vi "05T_Close_connection.vi"(11 "VISA":refnum<visa-resource-name>) -> ()   [LabVIEW 2013]
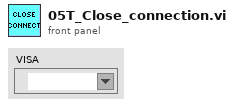
[diagram p1: front panel]
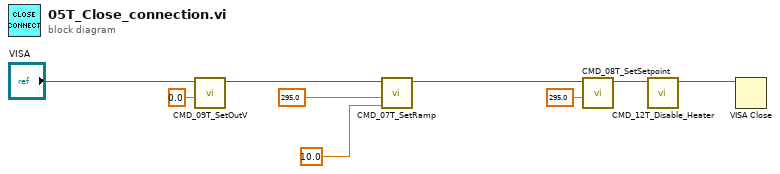
[diagram p0: block diagram]
diagram:
  n1 = call "CMD_09T_SetOutV.vi"("Voltage, d"=0.0, "VISA resource name"="VISA") -> ("VISA resource name out"=w3:refnum<visa-resource-name>)  [unwired: 9 in]
  n2 = call "CMD_07T_SetRamp.vi"("Ramp speed, K/min"=10.0, "Target, K"=295.0, "VISA resource name"=w3) -> ("VISA resource name out"=w4:refnum<visa-resource-name>)  [unwired: 8 in]
  n3 = call "CMD_08T_SetSetpoint.vi"("Setpoint, K"=295.0, "VISA resource name"=w4) -> ("VISA resource name out"=w7:refnum<visa-resource-name>)  [unwired: 9 in]
  n4 = call "CMD_12T_Disable_Heater.vi"("VISA resource name"=w7) -> ("VISA resource name out"=w6:refnum<visa-resource-name>)  [unwired: 10 in]
  n5 = VISA Close(VISA resource name=w6) -> ()  [unwired: 1 in, 1 out]
